vi "CRYFlatten results.vi"(11 "Result in":T1={"Name"="Test for Signal [L]", "Margin"=nan, "unit"="", "Verdict"=FALSE, "Limit"="", "Max/Min"="", "protected"=FALSE, "Step No."=0, "Test Info"="", "AutoProtect"=FALSE} {"Margin" format="%.2f"}) -> (3 "Flatten Result":string)   [LabVIEW 2013]
uses:
  Typedef Control/CRYResult Cluster.ctl
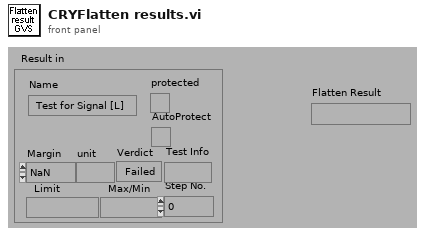
[diagram p1: front panel]
types:
  T1 = typedef "CRYResult Cluster.ctl" = cluster{"Name":string, "Margin":dbl, "unit":string, "Verdict":bool, "Limit":string, "Max/Min":string, "protected":bool, "Step No.":i32, "Test Info":string, "AutoProtect":bool}
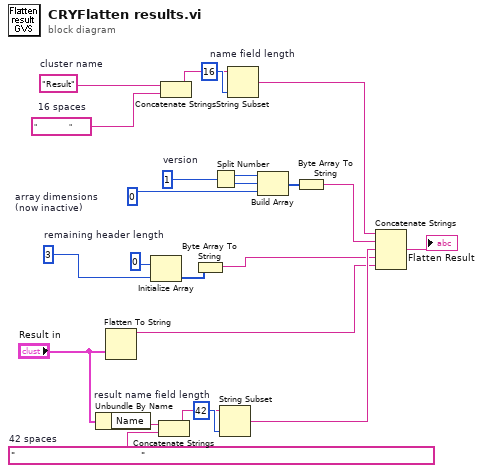
[diagram p0: block diagram]
diagram:
  w2 = "                                          "  # 42 spaces
  w8 = 42  # result name field length
  w10 = u8 0  # array dimensions (now inactive)
  w13 = 16  # name field length
  w14 = "                "  # 16 spaces
  w15 = "Result"  # cluster name
  w19 = 3  # remaining header length
  w23 = u16 1  # version
  n1 = Unbundle By Name("Result in") -> ("Name"=w9:string)
  n2 = Flatten To String(anything="Result in") -> (data string=w4:string)  [unwired: 3 in, 2 out]
  n3 = Initialize Array(u8 0, w19) -> (w6:u8[])
  n4 = Concatenate Strings(w9, w2) -> (w7:string)
  n5 = Concatenate Strings(w15, w14) -> (w12:string)
  n6 = Byte Array To String(unsigned byte array=w6) -> (string=w3:string)
  n7 = Split Number(x=w23) -> (hi(x)=w22:u8, lo(x)=w21:u8)
  n8 = String Subset(string=w7, length (rest)=w8) -> (substring=w5:string)  [unwired: 1 in]
  n9 = String Subset(string=w12, length (rest)=w13) -> (substring=w11:string)  [unwired: 1 in]
  n10 = Build Array(w22, w21, w10) -> (w18:u8[])
  n11 = Byte Array To String(unsigned byte array=w18) -> (string=w16:string)
  n12 = Concatenate Strings(w11, w16, w5, w3, w4) -> (→"Flatten Result":string)
